vi "MAIN - TLB` Springboard Tool.vi"() -> ()   [LabVIEW 2015, in "TLB` Springboard.lvlib"]
doc: "TLB Prime - Application Template 1.3.0.24\nNorm Kirchner, NI Systems Engineering - NI\nCopyright (c) 2014, NI"
uses:
  TLB` Springboard.lvlib
  Components/State Declaration.ctl
  Components/System Triggers.ctl
  <vilib>/Utility/error.llb/DialogTypeEnum.ctl
  <vilib>/NI/AMC/Read Termination Message.vi
  <vilib>/NI/AMC/Create Single Message.vi
  <vilib>/NI/AMC/Update Message Routing Info.vi
  <vilib>/NI/AMC/Create Multiple Messages.vi
  Components/TypeDef - SHIFTER - TLB` Springboard.ctl
  <vilib>/NI/AMC/Globals.vi
  <vilib>/NI/AMC/Send Message.vi
  Components/Dependencies.llb/TLB`_Dependencies.lvlib
  <vilib>/NI/AMC/AMC.lvlib
panel:
  in  "Add to Project":u16(ring) items=["< Create In New Project... >"]
  in  "Cancel":bool
  in  "Build":bool
  in  "New TLB Name":string
  in  "Destination Folder":path
  out "error out":errorcluster
  # "TLB` Springboard"
  # "Description"
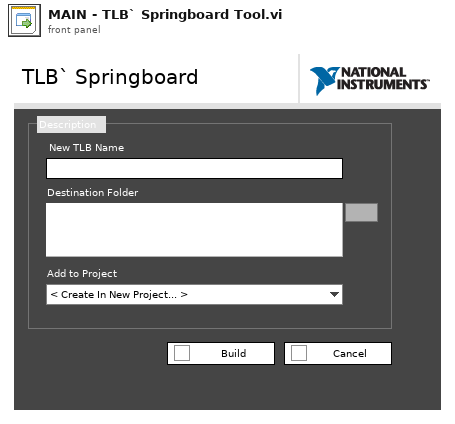
[diagram p1: front panel]
types:
  T1 = typedef "TLB` Springboard.lvlib/System Triggers.ctl" = enum16{"<None>", "Create New", "Cache User Parameters", "Close Application"}
  T2 = typedef "TLB` Springboard.lvlib/State Declaration.ctl" = enum16{"<Startup>", "Idle", "Creating", "<Shutdown>"}
  T3 = enum16{"Clear SR", "Set Display", "Set Shifter", "Initialize Events", "Init Q"}
  T4 = typedef "TLB` Springboard.lvlib/TypeDef - SHIFTER - TLB` Springboard.ctl" = cluster{"State":T2, "User Data":cluster{"New TLB Name":string, "Destination Folder":path, "Project Selection":u16}, "Display Data":cluster{"Active Item Tag":string}, "User Parameter Controls":refnum<vi>[], "Framework Data":cluster{"Exit Event":T5, "Terminate Error":errorcluster}, "Private Data":cluster{"Projects In Memory":refnum<vi>[], "Build Complete":bool}}
  T5 = typedef "TLB` Springboard.lvlib/TLB`_Dependencies.lvlib/Exit Event Ref.ctl" = refnum<user-event>
  T6 = typedef "AMC.lvlib/Message Queue.ctl" = refnum<queue>
  T7 = typedef "DialogTypeEnum.ctl" = enum16{"no dialog", "OK message", "continue or stop message", "auto error handling dialog", "OK message + warnings", "continue/stop + warnings"}
  T8 = enum8{"Enabled", "Disabled", "Disabled and Grayed Out"}
  T9 = enum32{"Invalid", "Standard", "Closed", "Hidden", "Minimized", "Maximized"}
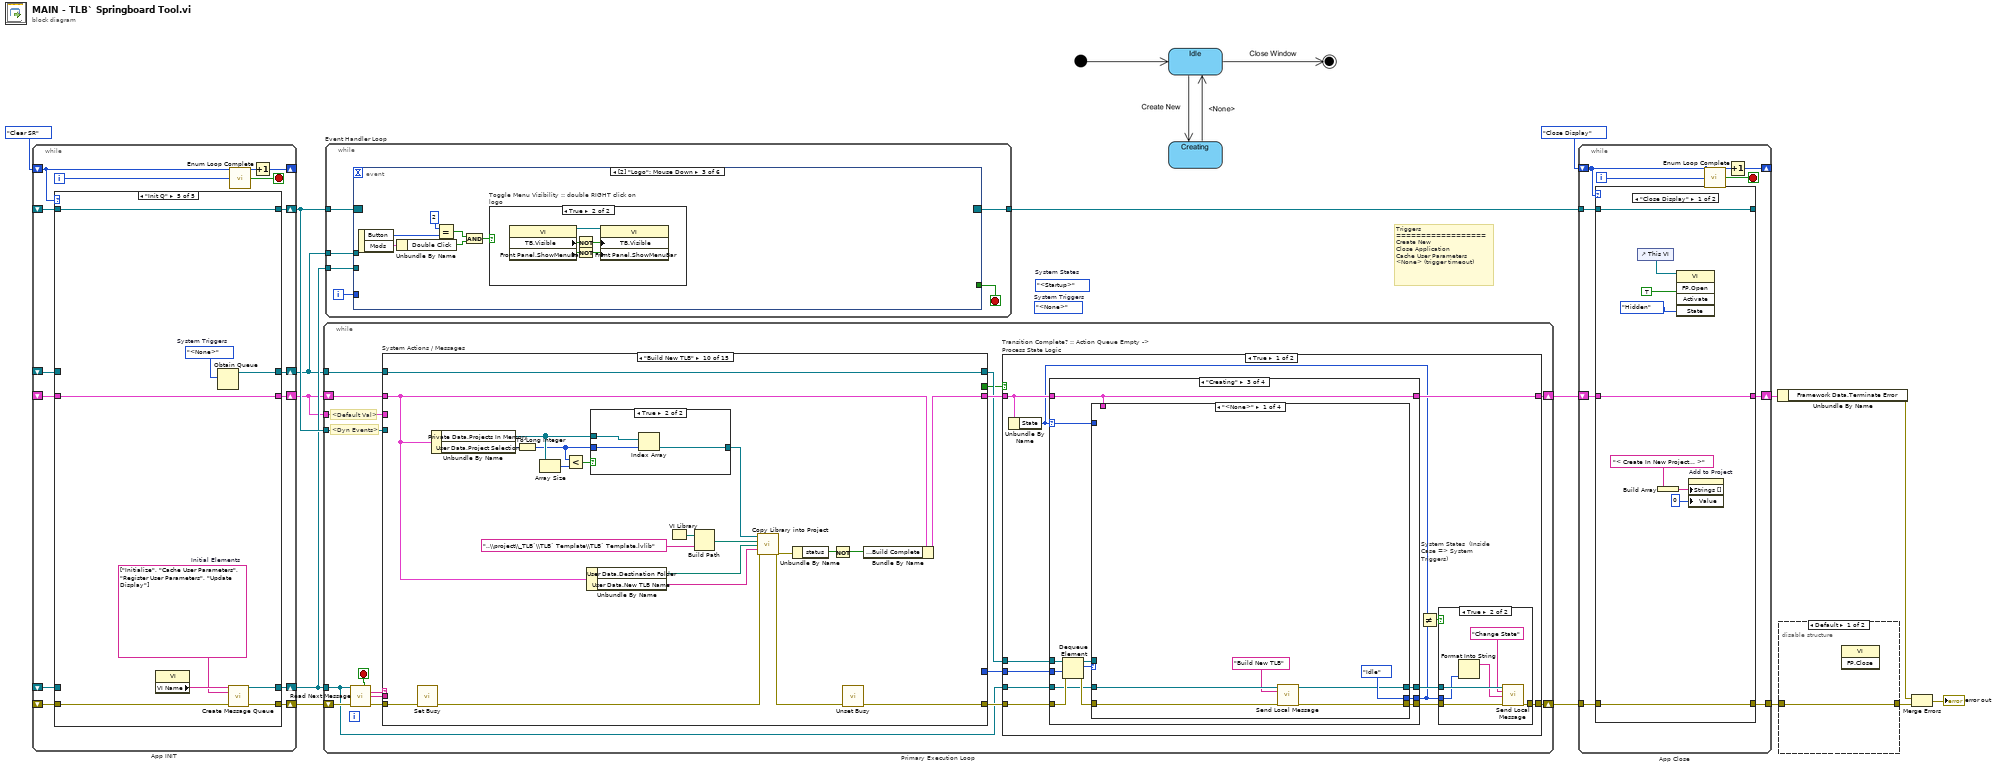
[diagram p0: block diagram]
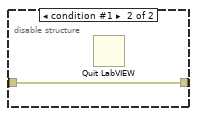
[diagram p2: hidden frame]
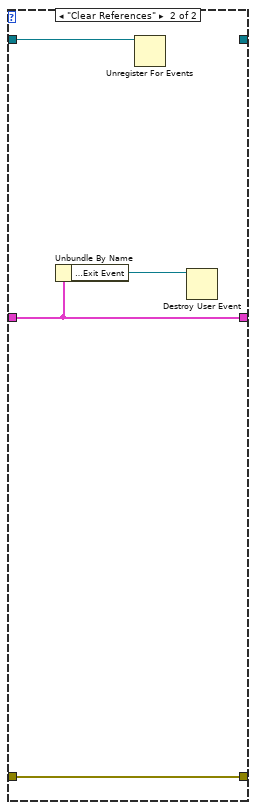
[diagram p3: hidden frame]
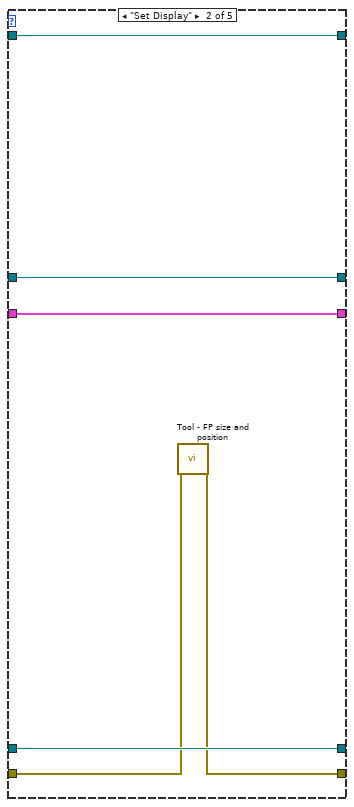
[diagram p5: hidden frame]
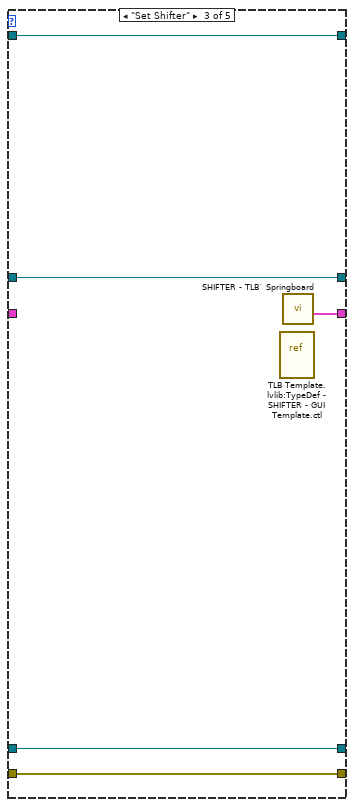
[diagram p6: hidden frame]
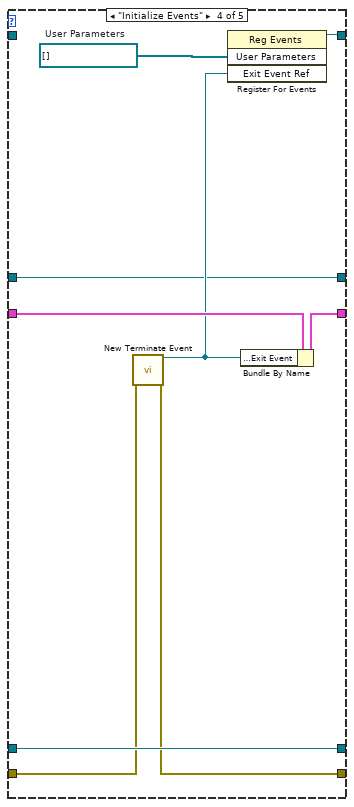
[diagram p7: hidden frame]
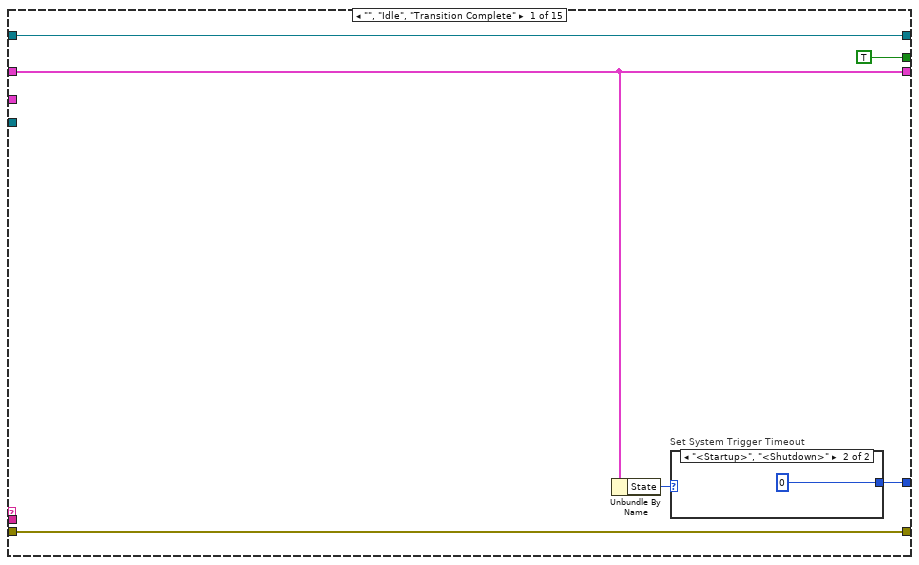
[diagram p8: hidden frame]
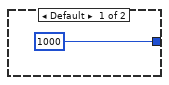
[diagram p9: hidden frame]
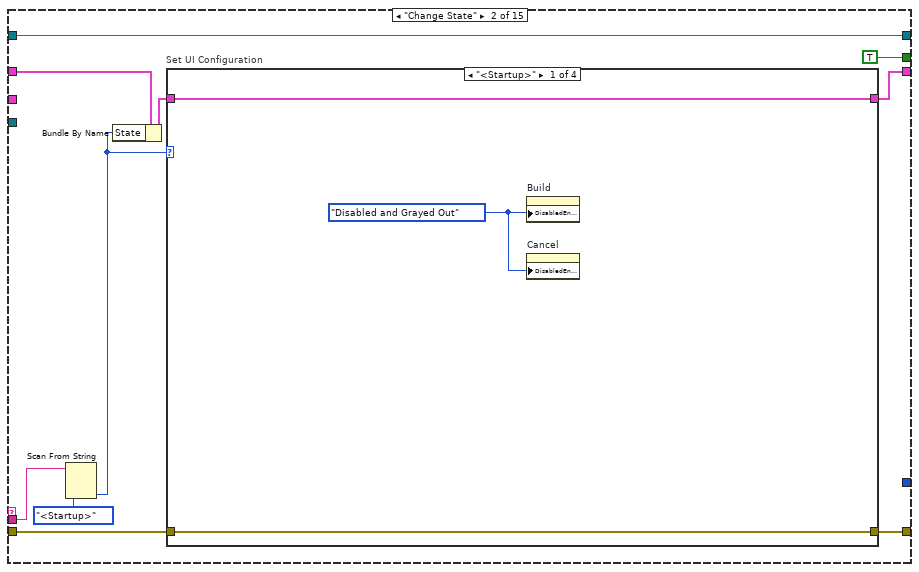
[diagram p10: hidden frame]
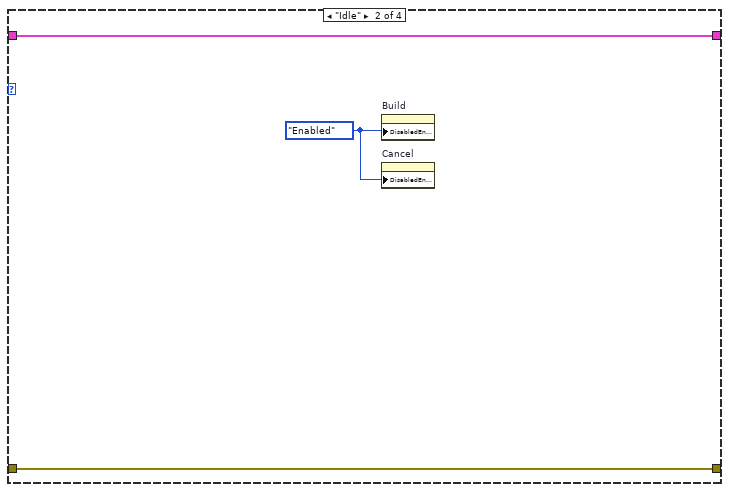
[diagram p11: hidden frame]
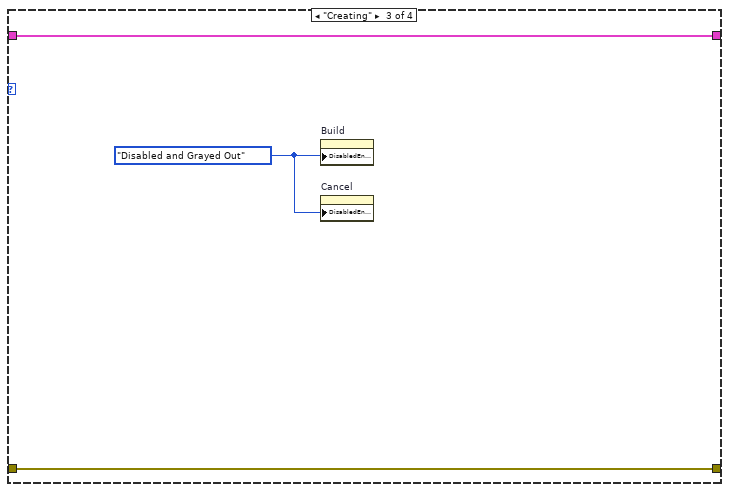
[diagram p12: hidden frame]
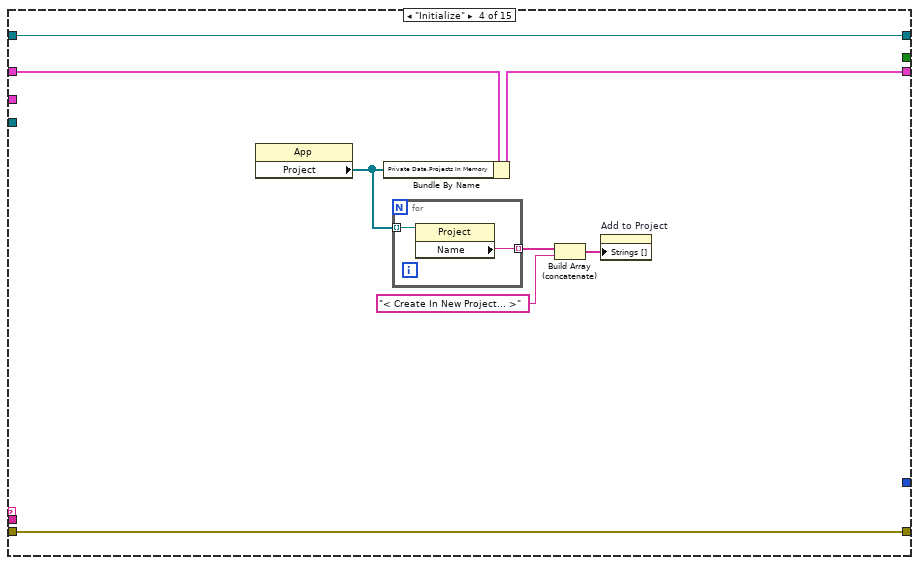
[diagram p15: hidden frame]
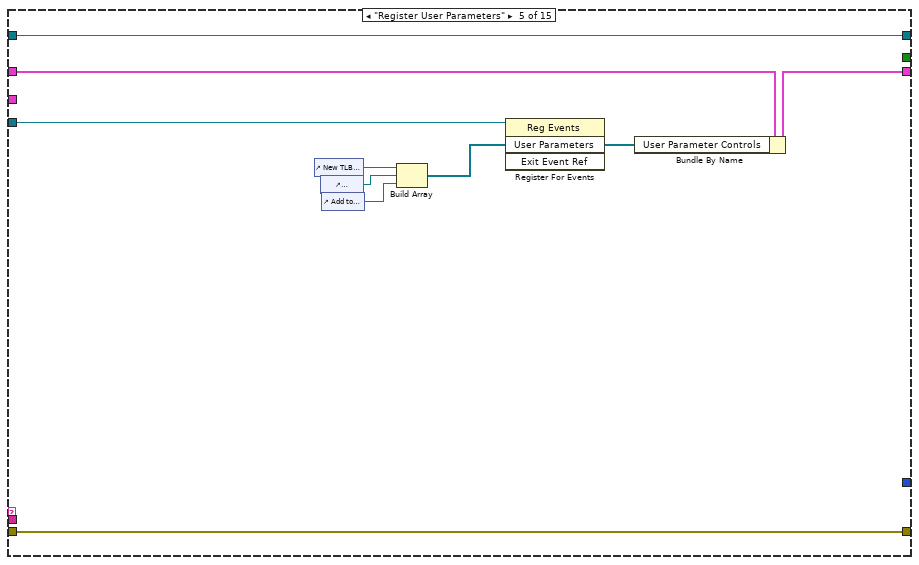
[diagram p16: hidden frame]
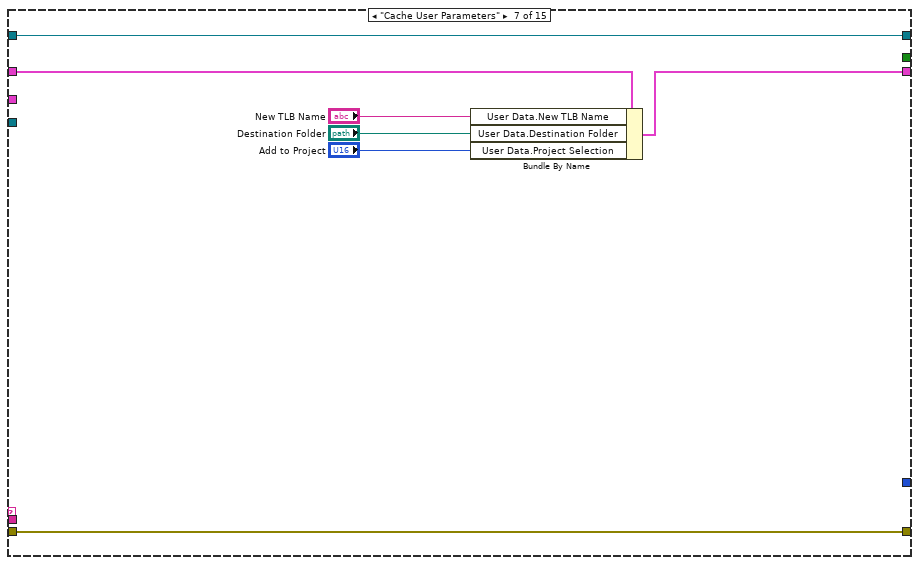
[diagram p18: hidden frame]
diagram:
  (unwired) System_Triggers."<None>"  # System Triggers
  (unwired) State_Declaration."<Startup>"  # System States
  # "Triggers\n==================\nCreate New\nClose Application\nCache User Parameters\n<None> (trigger timeout)"
  n1 = while "App INIT" {
    shift-right: [w23] -> _
    shift-left: T3."Clear SR" -> [w18]
    shift-right: [w29] -> w9
    shift-left: _ -> [w22]
    shift-right: [w26] -> w8
    shift-left: _ -> [w21]
    shift-right: [w28] -> w11
    shift-left: _ -> [w20]
    shift-right: [w27] -> w1
    shift-left: _ -> [w19]
    shift-right: [w17] -> w2
    shift-left: _ -> [w16]
    i -> [w24]
    stop <- w25 stop-if-true
    n2 = case shown="\"Init Q\"" w18 {
      tunnel: [_ w33 w40 w49 w55] -> w29
      tunnel: [_ w31 w39 w42 w53] -> w26
      tunnel: [_ w35 w36 w46 w57] -> w27
      tunnel: [_ w34 w38 w45 w58] -> w28
      tunnel: w22 -> [_ w33 w40 w49 _]
      tunnel: w21 -> [_ w32 w39 w43 w54]
      tunnel: w20 -> [_ w34 w38 _ w58]
      tunnel: w19 -> [_ w35 _ w47 w57]
      tunnel: [_ w30 w37 w41 w51] -> w17
      tunnel: w16 -> [_ w30 w37 w41 _]
      frame "Clear SR" {
      }
      frame "Set Display" {
        n3 = call "Tool - FP size and position.vi"("error in (no error)"=w32) -> ("error out"=w31:errorcluster)  [unwired: 7 in, 11 out]
      }
      frame "Set Shifter" {
        n4 = vi-ref "TLB Template.lvlib:TypeDef - SHIFTER - GUI Template.ctl"() -> ()  [unwired: 1 out]
        n5 = call "SHIFTER - TLB` Springboard.vi"() -> ("SHIFTER DATA"=w36:T4)  [unwired: 15 in]
      }
      frame "Initialize Events" {
        w48 = refnum<vi>[] []  # User Parameters
        n6 = call "New Terminate Event.vi"("error in (no error)"=w43) -> ("Exit Event Ref"=w44:T5, "error out"=w42:errorcluster)  [unwired: 13 in]
        n7 = register-events(w48, w44) -> (reference out=w45:refnum<event-registration>)  [unwired: 2 in, 1 out]
        n8 = Bundle By Name(cluster=w47, "Framework Data.Exit Event"=w44) -> (w46:T4)
      }
      frame "Init Q" {
        w50 = System_Triggers."<None>"  # System Triggers
        w52 = string[] ["Initialize", "Cache User Parameters", "Register User Parameters", "Update Display"]  # Initial Elements
        n9 = property class="VI"() -> ("VI Name"=w56:string)  [unwired: 2 in, 2 out]
        n10 = Obtain Queue(element data type=w50) -> (queue out=w51:refnum<queue>)  [unwired: 4 in, 2 out]
        n11 = call <vilib>:"Create Message Queue.vi"("message queue name"=w56, "initial message names"=w52, "error in"=w54) -> ("message queue out"=w55:T6, "error out"=w53:errorcluster)  [unwired: 11 in]
      }
    }
    n12 = call "Enum Loop Complete.vi"("Current State Enum"=w18, "Itteration"=w24) -> ("Loop Complete?"=w25:bool)  [unwired: 13 out]
    n13 = Increment(x=w18) -> (x+1=w23:T3)
  }
  n14 = while "Primary Execution Loop" {
    shift-right: [w65] -> w15
    shift-left: w8 -> [w72]
    shift-right: [w68] -> w14
    shift-left: w1 -> [w75]
    tunnel: w1 -> [w74]
    tunnel: w9 -> [w63]
    tunnel: w11 -> [w73]
    tunnel: w2 -> [w64]
    stop <- w70 stop-if-true
    # "<Dyn Events>"
    # "<Default Val>"
    n15 = call <vilib>:"Read Next Message.vi"("message queue in"=w63, "error in"=w72) -> ("exit process?"=w70:bool, "message name"=w69:string, "message value"=w60:string, "error out"=w71:errorcluster)  [unwired: 6 in, 4 out]
    n16 = case "System Actions / Messages" shown="\"Build New TLB\"" w69 {
      selector: w69 -> [_ _ _ _ _ _ _ _ _ _ _ _ _ _ w207]
      tunnel: [w81 w88 w107 w113 w126 w129 w134 w139 w142 w147 w170 w175 w197 w201 w211] -> w66
      tunnel: w71 -> [w81 w87 w107 w113 w126 w129 w134 w139 w142 w157 w170 w176 w197 w200 w212]
      tunnel: w75 -> [w76 w84 w106 w115 w125 w128 w136 w138 w141 w146 w169 w173 w196 w204 w213]
      tunnel: w74 -> [_ _ _ _ _ _ _ _ _ _ _ _ _ _ _]
      tunnel: [w76 w86 w106 w110 w124 w128 w135 w138 w141 w145 w169 w174 w196 w204 w213] -> w67
      tunnel: [w77 _ _ _ _ _ _ _ _ _ _ _ _ _ _] -> w59
      tunnel: w73 -> [_ _ _ _ w123 _ _ _ _ _ _ _ _ _ _]
      tunnel: [w79 w92 w105 w114 w122 w127 w133 w137 w140 w162 w168 w171 w195 w198 w205] -> w62
      tunnel: w64 -> [w79 w92 w105 w114 w122 w127 w133 w137 w140 w162 w168 w171 w195 w198 w205]
      tunnel: [TRUE TRUE _ _ _ _ _ _ _ _ _ _ _ _ _] -> w61
      tunnel: w60 -> [_ w91 _ _ _ _ _ _ _ _ _ _ _ _ _]
      frame "", "Idle", "Transition Complete" {
        n17 = Unbundle By Name(w76) -> ("State"=w78:T2)
        n18 = case "Set System Trigger Timeout" shown="\"<Startup>\", \"<Shutdown>\"" w78 {
          tunnel: [1000 0] -> w77
          frame Default {
          }
          frame "<Startup>", "<Shutdown>" {
          }
        }
      }
      frame "Change State" {
        n19 = Scan From String(input string=w91, default 1=State_Declaration."<Startup>" ("State")) -> (output 1=w89:T2)  [unwired: 3 in, 3 out]
        n20 = Bundle By Name(cluster=w84, "State"=w89) -> (w85:T4)
        n21 = case "Set UI Configuration" shown="\"<Startup>\"" w89 {
          tunnel: [w95 w99 w102 w104] -> w88
          tunnel: w87 -> [w95 w99 w102 w104]
          tunnel: [w96 w98 w101 w103] -> w86
          tunnel: w85 -> [w96 w98 w101 w103]
          frame "<Startup>" {
            w94 = T8."Disabled and Grayed Out" ("Disabled")
            n22 = property on="Build" class="Bool"("DisabledEnum"=w94) -> ()  [unwired: 2 in, 2 out]
            n23 = property on="Cancel" class="Bool"("DisabledEnum"=w94) -> ()  [unwired: 2 in, 2 out]
          }
          frame "Idle" {
            w97 = T8."Enabled" ("Disabled")
            n24 = property on="Build" class="Bool"("DisabledEnum"=w97) -> ()  [unwired: 2 in, 2 out]
            n25 = property on="Cancel" class="Bool"("DisabledEnum"=w97) -> ()  [unwired: 2 in, 2 out]
          }
          frame "Creating" {
            w100 = T8."Disabled and Grayed Out" ("Disabled")
            n26 = property on="Build" class="Bool"("DisabledEnum"=w100) -> ()  [unwired: 2 in, 2 out]
            n27 = property on="Cancel" class="Bool"("DisabledEnum"=w100) -> ()  [unwired: 2 in, 2 out]
          }
          frame "<Shutdown>" {
          }
        }
      }
      frame "/*********Initialize********/" {
      }
      frame "Initialize" {
        n28 = property class="App"() -> ("Project"=w109:refnum<vi>[])  [unwired: 2 in, 2 out]
        n29 = Bundle By Name(cluster=w115, "Private Data.Projects In Memory"=w109) -> (w110:T4)
        n30 = for {
          tunnel: w109 -> [w117] mode=indexing
          tunnel: [w116] -> w112 mode=indexing
          n31 = property class="Project"(reference=w117) -> ("Name"=w116:string)  [unwired: 1 in, 2 out]
        }
        n32 = Build Array (concatenate)(w112, "< Create In New Project... >") -> (w108:string[])
        n33 = property on="Add to Project" class="Ring (strict)"("Strings []"=w108) -> ()  [unwired: 2 in, 2 out]
      }
      frame "Register User Parameters" {
        n34 = control-ref of="New TLB Name"() -> (w120:refnum<vi>)
        n35 = control-ref of="Destination Folder"() -> (w118:refnum<vi>)
        n36 = control-ref of="Add to Project"() -> (w119:refnum<vi>)
        n37 = Build Array(w120, w118, w119) -> (w121:refnum<vi>[])
        n38 = register-events(reference=w123, w121) -> ()  [unwired: 2 in, 2 out]
        n39 = Bundle By Name(cluster=w125, "User Parameter Controls"=w121) -> (w124:T4)
      }
      frame "/*********Display Updates********/" {
      }
      frame "Cache User Parameters" {
        n40 = Bundle By Name(cluster=w136, "User Data.New TLB Name"="New TLB Name", "User Data.Destination Folder"="Destination Folder", "User Data.Project Selection"="Add to Project") -> (w135:T4)
      }
      frame "Update Display" {
      }
      frame "/*********Primary Execution********/" {
      }
      frame "Build New TLB" {
        n41 = call <vilib>:"Set Busy.vi"("error in (no error)"=w157) -> ("error out"=w152:errorcluster)  [unwired: 9 in, 1 out]
        n42 = Unbundle By Name(w146) -> ("Private Data.Projects In Memory"=w159:refnum<vi>[], "User Data.Project Selection"=w161:u16)
        n43 = To Long Integer(number=w161) -> (32bit integer=w143:i32)
        n44 = Array Size(array=w159) -> (size(s)=w160:i32)
        n45 = Less?(x=w143, y=w160) -> (x < y?=w158:bool)
        n46 = Unbundle By Name(w146) -> ("User Data.Destination Folder"=w154:path, "User Data.New TLB Name"=w153:string)
        n47 = case shown="True" w158 {
          tunnel: w143 -> [_ w167]
          tunnel: w159 -> [_ w166]
          tunnel: [w163 w165] -> w156
          frame False {
            n48 = invoke class="App" method="Project.New"() -> ("Project:New"=w164:refnum<vi>)  [unwired: 3 in, 2 out]
            n49 = invoke class="Project" method="Open Window"(reference=w164) -> (reference out=w163:refnum<vi>)  [unwired: 2 in, 2 out]
          }
          frame True {
            n50 = Index Array(array=w166, index=w167) -> (element=w165:refnum<vi>)
          }
        }
        n51 = VI Library() -> (path=w151:path)
        n52 = Build Path(base path=w151, name or relative path="..\\project\\_TLB`\\TLB` Template\\TLB` Template.lvlib") -> (appended path=w155:path)
        n53 = call "Copy Library into Project.vi"("Project"=w156, "Library Path"=w155, "Destination Folder"=w154, "New TLB Name"=w153, "error in"=w152) -> ("error out"=w149:errorcluster)  [unwired: 10 in]
        n54 = Unbundle By Name(w149) -> ("status"=w148:bool)
        n55 = Not(x=w148) -> (.not. x?=w144:bool)
        n56 = call <vilib>:"Unset Busy.vi"("error in (no error)"=w149) -> ("error out"=w147:errorcluster)  [unwired: 10 in]
        n57 = Bundle By Name(cluster=w146, "Private Data.Build Complete"=w144) -> (w145:T4)
      }
      frame "/*********Shutdown********/" {
      }
      frame "Error" {
        n58 = Unbundle By Name(w173) -> ("State"=w172:T2)
        n59 = case shown="Default" w172 {
          tunnel: w176 -> [w184]
          tunnel: [w183] -> w175
          tunnel: w173 -> [w180]
          tunnel: [w179] -> w174
          tunnel: w171 -> [w177]
          frame Default {
            n60 = call <vilib>:"General Error Handler CORE.vi"("type of dialog (OK msg:1)"=DialogTypeEnum."auto error handling dialog", "error in (no error)"=w184) -> ("stop event propagated"=w182:bool, "error out"=w178:errorcluster)  [unwired: 12 out]
            n61 = case "User Chose to Stop and Not Continue\nFALSE = Continue: CLEAR ERRORS" shown="True" w182 {
              tunnel: [w185 w189] -> w183
              tunnel: w178 -> [w186 w192]
              tunnel: w180 -> [w187 w194]
              tunnel: [w187 w193] -> w179
              tunnel: w177 -> [_ w190]
              frame False {
                n62 = call <vilib>:"Clear Errors.vi"("error in (no error)"=w186) -> ("error out"=w185:errorcluster)  [unwired: 1 in, 5 out]
              }
              frame True {
                n63 = call <vilib>:"Clear Errors.vi"("error in (no error)"=w192) -> ("error out"=w188:errorcluster)  [unwired: 1 in, 5 out]
                n64 = Bundle By Name(cluster=w194, "Framework Data.Terminate Error"=w192) -> (w193:T4)
                n65 = Enqueue Element(queue=w190, element=System_Triggers."Close Application", error in (no error)=w188) -> (error out=w189:errorcluster)  [unwired: 1 in, 2 out]
              }
            }
          }
        }
      }
      frame "Close Window" {
      }
      frame "Exit" {
        w199 = refnum<class> refnum  # event data
        # "Don't wire 'Error In'\nMust Execute Regardless"
        n66 = Unbundle By Name(w204) -> ("Framework Data.Exit Event"=w203:T5)
        n67 = Generate User Event(user event=w203, event data cluster=w199) -> (error out=w202:errorcluster)  [unwired: 2 in, 1 out]
        n68 = Merge Errors(w202, w200) -> (w201:errorcluster)
      }
      frame Default {
        w209 = 1 items=["No error", "Argument error", "Memory is full", "Out of zone", "End of file", "File already open", "Generic file I/O error", "File not found", "File permission error", "Disk is full", "Duplicate path", "Too many files open", "System feature not enabled", "Resource file not found", "Cannot add resource", "Resource not found", "Image not found", "Image memory error", "Pen does not exist", "Config type invalid", "Config token not found", "Config parse error", "Config memory error", "Bad external code format", "Bad external code offset", "External code not present", "Null window", "Destroy window error", "Null menu", "Print aborted", "Bad print record", "Print driver error", "Windows error during printing", "Memory error during printing", "Print dialog error", "Generic print error", "Invalid device refnum", "Device not found", "Device parameter error", "Device unit error", "Cannot open device", "Device call aborted", "Generic error", "Cancelled by user", "Object ID too low", "Object ID too high", "Object not in heap", "Unknown heap", "Unknown object (invalid DefProc)", "Unknown object (DefProc not in table)", "Message out of range", "Invalid (null) method", "Unknown message", "Manager call not supported", "Bad address", "Network operation in progress", "Network operation timed out", "Connection is busy", "Network attribute not supported", "Network error", "Address in use", "System out of memory", "Connection aborted", "Connection refused", "Not connected", "Already connected", "Connection closed", "Initialization error (interapplication manager)", "Bad occurrence", "Wait on unbound occurrence handler", "Occurrence queue overflow", "Datalog type conflict", "Unused", "Unrecognized type (interapplication manager)", "Memory corrupt", "Failed to make temporary DLL", "Old CIN version", "Drag socket not found", "Failed to load drop-object", "Failed to register OLE object", "Failed to release OLE object", "Format specifier type mismatch", "Unknown format specifier", "Too few format specifiers", "Too many format specifiers", "Scan failed", "Newer CIN version", "Error converting to variant", "Runtime menu error", "Password tampered", "Variant attribute not found", "Incompatible variant data type", "Event data is not available", "Event Store is not present", "Occurrence is not found", "Event Queue is not created", "Event info is not available", "Refnum passed is NULL", "Error retrieving Class GUID", "Error retrieving CoClass GUID", "Error retrieving TypeLib GUID.", "Bad built application magic bytes.", "Specific driver is different from the specific driver associated with the Logical Name.", "There is no session opened to the class driver.", "Max Error", "MAX - Error with config objects", "MAX - Error loading configuration", "MAX - Group not supported"]
        w210 = TRUE  # status
        n69 = Format Into String(format string="DEVELOPER ERROR:\nImproper State Requested\n================\nState {%s} does not exist within this architecture\n\nCheck for spelling and case errors" ("source"), w207) -> (resulting string=w208:string)  [unwired: 2 in, 1 out]
        n70 = Bundle By Name(cluster=w212, "status"=w210, "code"=w209, "source"=w208) -> (w211:errorcluster)
      }
    }
    n71 = case "Transition Complete? :: Action Queue Empty -> Process State Logic" shown="True" w61 {
      tunnel: [w225 w331] -> w68
      tunnel: w67 -> [w215 w331]
      tunnel: w66 -> [w224 w330]
      tunnel: w63 -> [w223 _]
      tunnel: [w219 w330] -> w65
      tunnel: w62 -> [w222 _]
      tunnel: w59 -> [w216 _]
      frame True {
        n72 = Unbundle By Name(w215) -> ("State"=w214:T2)
        n73 = case "System States  (Inside Case => System Triggers)" shown="\"Creating\"" w214 {
          selector: w214 -> [_ w250 w280 _]
          tunnel: [w241 w249 w290 w321] -> w225
          tunnel: w215 -> [w241 w249 w290 w321]
          tunnel: w224 -> [w235 w254 w284 w315]
          tunnel: w223 -> [w233 w252 w282 w313]
          tunnel: [w240 w259 w289 w320] -> w220
          tunnel: w222 -> [w243 w247 w291 w323]
          tunnel: [w239 w258 w288 w319] -> w221
          tunnel: [w238 w257 w287 w318] -> w218
          tunnel: w216 -> [w237 w255 w285 w317]
          frame "<Startup>" {
            n74 = Dequeue Element(queue=w243, timeout in ms (-1)=w237, error in (no error)=w235) -> (queue out=w236:refnum<queue>, element=w242:T1, error out=w234:errorcluster)  [unwired: 1 out]
            n75 = case shown="\"<None>\", Default" w242 {
              tunnel: w241 -> [_]
              tunnel: [w245] -> w240
              tunnel: w234 -> [w245]
              tunnel: w233 -> [w246]
              tunnel: [w246] -> w239
              tunnel: [State_Declaration."Idle" ("State")] -> w238
              tunnel: w236 -> [_]
              frame "<None>", Default {
              }
            }
          }
          frame "Idle" {
            n76 = Dequeue Element(queue=w247, timeout in ms (-1)=w255, error in (no error)=w254) -> (queue out=w251:refnum<queue>, element=w256:T1, error out=w253:errorcluster)  [unwired: 1 out]
            n77 = Unbundle By Name(w249) -> ("Private Data.Build Complete"=w248:bool)
            n78 = case shown="\"Create New\"" w256 {
              tunnel: w249 -> [_ _ _ _ _]
              tunnel: [w262 w266 w269 w272 w276] -> w259
              tunnel: w253 -> [w262 w266 w269 w272 w279]
              tunnel: w252 -> [w263 w265 w270 w273 w278]
              tunnel: [w263 w265 w270 w273 w277] -> w258
              tunnel: [State_Declaration."Idle" ("State") State_Declaration."Creating" ("State") State_Declaration."<Shutdown>" ("State") State_Declaration."Idle" ("State") w274] -> w257
              tunnel: w251 -> [_ _ _ _ _]
              tunnel: w250 -> [_ _ _ _ w274]
              frame "<None>" {
              }
              frame "Create New" {
              }
              frame "Close Application" {
              }
              frame Default {
              }
              frame "Cache User Parameters" {
                n79 = call <vilib>:"Send Local Message.vi"("message queue in"=w278, "message name"="Cache User Parameters" ("Message Name"), "error in"=w279) -> ("message queue out"=w277:T6, "error out"=w276:errorcluster)  [unwired: 10 in, 1 out]
              }
            }
            n80 = case shown="True" w248 {
              tunnel: w247 -> [_ w260]
              frame False {
              }
              frame True {
                n81 = Enqueue Element(queue=w260, element=System_Triggers."Close Application" ("System Triggers")) -> ()  [unwired: 2 in, 3 out]
              }
            }
          }
          frame "Creating" {
            n82 = Dequeue Element(queue=w291, timeout in ms (-1)=w285, error in (no error)=w284) -> (queue out=w281:refnum<queue>, element=w286:T1, error out=w283:errorcluster)  [unwired: 1 out]
            n83 = case shown="\"<None>\"" w286 {
              tunnel: w290 -> [_ _ _ _]
              tunnel: [w295 w300 w304 w308] -> w289
              tunnel: w283 -> [w296 w303 w304 w309]
              tunnel: w282 -> [w294 w302 w305 w307]
              tunnel: [w293 w301 w305 w307] -> w288
              tunnel: [State_Declaration."Idle" ("State") w298 State_Declaration."Creating" ("State") State_Declaration."Idle" ("State")] -> w287
              tunnel: w281 -> [_ _ _ w311]
              tunnel: w280 -> [_ w298 _ _]
              frame "<None>" {
                n84 = call <vilib>:"Send Local Message.vi"("message queue in"=w294, "message name"="Build New TLB" ("Message Name"), "error in"=w296) -> ("message queue out"=w293:T6, "error out"=w295:errorcluster)  [unwired: 10 in, 1 out]
              }
              frame "Cache User Parameters" {
                n85 = call <vilib>:"Send Local Message.vi"("message queue in"=w302, "message name"="Cache User Parameters" ("Message Name"), "error in"=w303) -> ("message queue out"=w301:T6, "error out"=w300:errorcluster)  [unwired: 10 in, 1 out]
              }
              frame Default {
              }
              frame "Close Application" {
                n86 = Enqueue Element(queue=w311, element=System_Triggers."Close Application" ("System Triggers"), error in (no error)=w309) -> (error out=w308:errorcluster)  [unwired: 1 in, 2 out]
              }
            }
          }
          frame "<Shutdown>" {
            n87 = Dequeue Element(queue=w323, timeout in ms (-1)=w317, error in (no error)=w315) -> (queue out=w316:refnum<queue>, element=w322:T1, error out=w314:errorcluster)  [unwired: 1 out]
            n88 = case shown="\"<None>\", Default" w322 {
              tunnel: w321 -> [_]
              tunnel: [w324] -> w320
              tunnel: w314 -> [w326]
              tunnel: w313 -> [w327]
              tunnel: [w325] -> w319
              tunnel: [State_Declaration."<Shutdown>" ("State")] -> w318
              tunnel: w316 -> [_]
              frame "<None>", Default {
                n89 = call <vilib>:"Send Local Messages.vi"("message queue in"=w327, "message names"=string[] ["Exit"], "error in"=w326) -> ("message queue out"=w325:T6, "error out"=w324:errorcluster)  [unwired: 10 in, 1 out]
              }
            }
          }
        }
        n90 = Not Equal?(x=w214, y=w218) -> (x != y?=w217:bool)
        n91 = case shown="True" w217 {
          tunnel: w221 -> [_ w232]
          tunnel: w220 -> [w226 w231]
          tunnel: [w226 w230] -> w219
          tunnel: w218 -> [_ w228]
          frame False {
          }
          frame True {
            n92 = Format Into String(w228) -> (resulting string=w227:string)  [unwired: 3 in, 1 out]
            n93 = call <vilib>:"Send Local Message.vi"("message queue in"=w232, "message name"="Change State" ("Message Name"), "message value"=w227, "error in"=w231) -> ("error out"=w230:errorcluster)  [unwired: 9 in, 2 out]
          }
        }
      }
      frame False {
      }
    }
  }
  n94 = while "Event Handler Loop" {
    tunnel: w11 -> [w336]
    tunnel: w9 -> [w335]
    tunnel: [w334] -> w13
    tunnel: w2 -> [w332]
    i -> [w333]
    stop <- w337 stop-if-true
    n95 = event shown="[2] \"Logo\": Mouse Down" {
      selector: w336 -> [_ _ _ _ _ _]
      dyn-events: [_ _ _ _ _ _] -> w334
      timeout: _ -> [_ _ _ _ _ _]
      tunnel: [_ _ _ TRUE ("NewVal") _ _] -> w337
      tunnel: w335 -> [_ _ _ _ _ _]
      tunnel: w333 -> [_ _ _ _ _ _]
      tunnel: w332 -> [w339 w342 _ w355 w359 w361]
      event Panel Close? {
        w340 = TRUE  # Discard?
        n96 = event-data() -> ()  [unwired: 2 out]
        n97 = Enqueue Element(queue=w339, element=System_Triggers."Close Application") -> ()  [unwired: 2 in, 3 out]
        n98 = event-data("Discard?"=w340) -> ()  [unwired: 1 in, 1 out]
      }
      event "Cancel": Value Change {
        n99 = event-data() -> ()  [unwired: 4 out]
        n100 = Enqueue Element(queue=w342, element=System_Triggers."Close Application") -> ()  [unwired: 2 in, 3 out]
      }
      event Mouse Down {
        n101 = event-data() -> ("Button"=w347:u16, "Mods"=w348:cluster{"Double Click":bool, "Menu Key":bool})  [unwired: 1 out]
        n102 = Unbundle By Name(w348) -> ("Double Click"=w344:bool)
        n103 = Equal?(x=u16 2, y=w347) -> (x = y?=w345:bool)
        n104 = And(x=w345, y=w344) -> (x .and. y?=w343:bool)
        n105 = case "Toggle Menu Visibility :: double RIGHT click on logo" shown="True" w343 {
          frame False {
          }
          frame True {
            n106 = property class="VI"() -> (reference out=w353:refnum<vi>, "TB.Visible"=w351:bool, "Front Panel.ShowMenuBar"=w350:bool)  [unwired: 2 in, 1 out]
            n107 = Not(x=w351) -> (.not. x?=w352:bool)
            n108 = Not(x=w350) -> (.not. x?=w349:bool)
            n109 = property class="VI"(reference=w353, "TB.Visible"=w352, "Front Panel.ShowMenuBar"=w349) -> ()  [unwired: 1 in, 2 out]
          }
        }
      }
      event User Event {
        w354 = System_Triggers."Close Application"  # System Triggers
        n110 = event-data() -> ()  [unwired: 2 out]
        n111 = Enqueue Element(queue=w355, element=w354) -> ()  [unwired: 2 in, 3 out]
      }
      event Value Change {
        n112 = event-data() -> ()  [unwired: 2 out]
        n113 = Enqueue Element(queue=w359, element=System_Triggers."Cache User Parameters") -> (queue out=w358:refnum<queue>)  [unwired: 2 in, 2 out]
        n114 = event "use this event case to register a SPEICIFIC 'User Parameter' for a SPECIFIC action" shown="[0] Timeout" {
          selector: _ -> [_]
          dyn-events: _ -> [_]
          timeout: 0 -> [_]
          tunnel: w358 -> [_]
          event Timeout {
            n115 = event-data() -> ()  [unwired: 1 in, 1 out]
          }
        }
      }
      event "Build": Value Change {
        n116 = event-data() -> ()  [unwired: 4 out]
        n117 = Enqueue Element(queue=w361, element=System_Triggers."Create New") -> ()  [unwired: 2 in, 3 out]
      }
    }
  }
  n118 = while "App Close" {
    shift-right: [w369] -> _
    shift-left: enum16{"Close Display", "Clear References"}."Close Display" -> [w368]
    tunnel: w13 -> [w366]
    tunnel: w15 -> [w367]
    tunnel: [w364] -> w7
    shift-right: [w363] -> w5
    shift-left: w14 -> [w365]
    i -> [w370]
    stop <- w371 stop-if-true
    n119 = case shown="\"Close Display\"" w368 {
      tunnel: [w379 w384] -> w364
      tunnel: [w378 w383] -> w363
      tunnel: [w380 _] -> _
      tunnel: w367 -> [w379 w384]
      tunnel: w366 -> [w380 w381]
      tunnel: w365 -> [w378 w383]
      frame "Close Display" {
        n120 = control-ref of="This VI"() -> (w372:refnum<vi>)
        n121 = Build Array("< Create In New Project... >") -> (w377:string[])
        n122 = invoke class="VI" method="FP.Open"(reference=w372, "Activate"=TRUE ("Activate?"), "State"=T9."Hidden") -> ()  [unwired: 2 in, 5 out]
        n123 = property on="Add to Project" class="Ring (strict)"("Strings []"=w377, "Value"=u16 0) -> ()  [unwired: 2 in, 2 out]
      }
      frame "Clear References" {
        n124 = Unbundle By Name(w383) -> ("Framework Data.Exit Event"=w382:T5)
        n125 = Unregister For Events(event registration refnum=w381) -> ()  [unwired: 1 in, 1 out]
        n126 = Destroy User Event(user event=w382) -> ()  [unwired: 1 in, 1 out]
      }
    }
    n127 = call "Enum Loop Complete.vi"("Current State Enum"=w368, "Itteration"=w370) -> ("Loop Complete?"=w371:bool)  [unwired: 13 out]
    n128 = Increment(x=w368) -> (x+1=w369:enum16{"Close Display", "Clear References"})
  }
  n129 = Unbundle By Name(w5) -> ("Framework Data.Terminate Error"=w3:errorcluster)
  n130 = disable-structure shown="Default" {
    disable-tunnel: [w385 w386] -> w4
    disable-tunnel: w7 -> [w385 w386]
    frame condition #0 (active) {
      n131 = invoke class="VI" method="FP.Close"() -> ()  [unwired: 3 in, 3 out]
    }
    frame condition #1 {
      n132 = Quit LabVIEW() -> ()  [unwired: 1 in]
    }
  }
  n133 = Merge Errors(w3, w4) -> (→"error out":errorcluster)
